vi "Read HDI-on-BBM Fiducials.vi"(8 "error in":errorcluster, 9 "Slot":u32, 10 "Chuck":u32, 11 "CameraTool in":refnum<class "CameraTool Class.lvclass">) -> (0 "error out":errorcluster, 3 "CameraTool out":refnum<class "CameraTool Class.lvclass">)   [LabVIEW 2011, in "CameraTool Class.lvclass"]
uses:
  CameraTool Class.lvclass
  WorkTable Class/WorkTable Class.lvclass
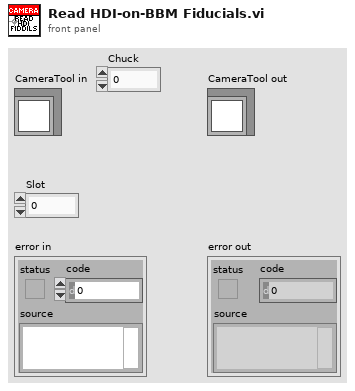
[diagram p1: front panel]
types:
  T1 = typedef "Worktable_BBM Slot.ctl" = cluster{"BBM Slot State":enum16{"Empty", "Unglued", "Stamped", "PartOnTop", "Weighted", "Unpotted", "Potted"}, "BBM Type":enum16{"BBM", "GlassSlide"}, "HDI Type":enum16{"HDI", "Polyimide"}, "Vacuum Channel":u8, "Location/Orientation BBM":T2, "Location/Orientation HDI":T2}
  T2 = typedef "Position_Orientation.ctl" = cluster{"Center":refnum<class "Vec3d Class.lvclass">, "Orientation":refnum<class "Orient3d Class.lvclass">}
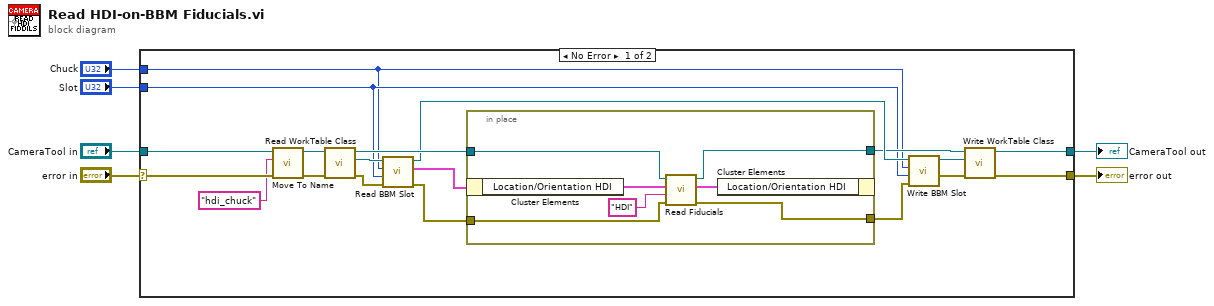
[diagram p0: block diagram]
diagram:
  n1 = case shown="No Error" "error in" {
    selector: "error in" -> [w16 w34]
    tunnel: [w17 w34] -> w2
    tunnel: [w18 w33] -> w3
    tunnel: "CameraTool in" -> [w19 w33]
    tunnel: "Slot" -> [w8 _]
    tunnel: "Chuck" -> [w7 _]
    frame No Error {
      n2 = call-dynamic "Move To Name.vi"("error in"=w16, "Destination Name"="hdi_chuck" ("format string"), "Gantry in"=w19) -> ("error out"=w25:errorcluster, "Gantry out"=w24:refnum<class "CameraTool Class.lvclass">)  [unwired: 7 in]
      n3 = call-dynamic "Read WorkTable Class.vi"("error in"=w25, "Gantry Class in"=w24) -> ("error out"=w22:errorcluster, "WorkTable Class.lvclass"=w23:refnum<class "WorkTable Class.lvclass">, "Gantry Class out"=w13:refnum<class "CameraTool Class.lvclass">)  [unwired: 7 in]
      n4 = call-dynamic "Read BBM Slot.vi"("error in (no error)"=w22, "Slot Number"=w8, "Chuck Number"=w7, "WorkTable Class in"=w23) -> ("error out"=w14:errorcluster, "BBM Slot"=w12:T1, "WorkTable Class out"=w11:refnum<class "WorkTable Class.lvclass">)  [unwired: 5 in]
      n5 = in-place {
        in-place-border: w14 -> [w28]
        in-place-border: w13 -> [w30]
        in-place-border: [w29] -> w10
        in-place-border: [w27] -> w9
        n6 = in-place-cluster #1(w12) -> ("Location/Orientation HDI"=w32:T2)
        n7 = call-dynamic "Read Fiducials.vi"("error in"=w28, "Part Name"="HDI", "Location/Orientation in"=w32, "CameraTool in"=w30) -> ("error out"=w27:errorcluster, "Location/Orientation out"=w31:T2, "CameraTool out"=w29:refnum<class "CameraTool Class.lvclass">)  [unwired: 5 in]
        n8 = in-place-cluster #1("Location/Orientation HDI"=w31) -> ()  [unwired: 1 out]
      }
      n9 = call-dynamic "Write BBM Slot.vi"("error in (no error)"=w9, "Slot Number"=w8, "Chuck Number"=w7, "WorkTable Class in"=w11) -> ("error out"=w20:errorcluster, "WorkTable Class out"=w21:refnum<class "WorkTable Class.lvclass">)  [unwired: 6 in]
      n10 = call-dynamic "Write WorkTable Class.vi"("error in (no error)"=w20, "WorkTable Class.lvclass"=w21, "Gantry Class in"=w10) -> ("error out"=w17:errorcluster, "Gantry Class out"=w18:refnum<class "CameraTool Class.lvclass">)  [unwired: 7 in]
    }
    frame Error {
    }
  }
  "error out" <- w2
  "CameraTool out" <- w3
